vi "Overlay selected point in a miniscan.vi"(8 "error in":errorcluster, 9 "Data reference":refnum<data-value>) -> (0 "error out":errorcluster)   [LabVIEW 2017]
uses:
  xcontrol/Interface VIs/Interface typedefs/Interface-Data array.ctl
  xcontrol/Interface VIs/Interface typedefs/Interface-Data format definition.ctl
  xcontrol/Typedefs/Xctl-XY data type definition.ctl
  xcontrol/Typedefs/Xctrl-ROI type enum.ctl
  Typedefs/Get-Set-Clear Control.ctl
  Global variables/gl_Functional Imaging-Global variables.vi
  xcontrol/XGrapher.xctl
panel:
  in  "Miniscan point overlay colour":u32(colorbox)=16711907
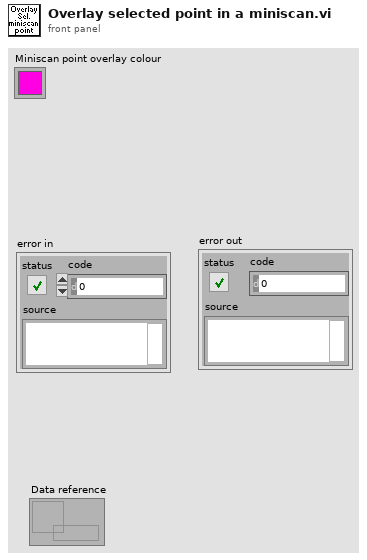
[diagram p1: front panel]
types:
  T1 = typedef "Get-Set-Clear Control.ctl" = enum16{"Get", "Set", "Clear"}
  T2 = typedef "Functional Imging UI Refs.ctl" = cluster{"Menu ref":refnum<k9>, "Image control":refnum<vi>, "VI ref":refnum<vi>, "XGrapher":refnum<vi>, "Smoothing":refnum<vi>, "POI Averaging":refnum<vi>, "Normalize":refnum<vi>, "POI data points in each trial":refnum<vi>, "Channel":refnum<vi>, "Experiment data folder path":refnum<vi>, "[ROI vis]":refnum<vi>, "[Groups] visbl":T3, "Group Name":refnum<vi>, "POI index":refnum<vi>, "Trial No.":refnum<vi>, "Intensity Zoom":refnum<vi>, "Trial Cursor Enabled":refnum<vi>, "Number of Trials (ind 1)":refnum<vi>, "Number of Trials (ind 2)":refnum<vi>, "MiniScans Available":refnum<vi>, "POI Available":refnum<vi>, "Defer graph updates":refnum<vi>, "Waveform selector":refnum<vi>, "#of selected POI":refnum<vi>, "#of selected MiniScans":refnum<vi>, "#of selected groups":refnum<vi>, "Max Z-Projection":refnum<vi>, "Z-Plane Selector":refnum<vi>, "Index of miniscan point to visualise":refnum<vi>, "ROI vis. mode":refnum<vi>, "Total # of points":refnum<vi>, "Index of group clicked on":refnum<vi>, "Pane 1":refnum<vi>, "Pane 2":refnum<vi>, "Pane 3":refnum<vi>, "Pane 4":refnum<vi>, "Pane 5":refnum<vi>, "Pane 6":refnum<vi>, "Deselect all ROI":refnum<vi>, "Deselect all groups":refnum<vi>}
  T3 = typedef "Groups array referecne.ctl" = refnum<vi>
  T4 = typedef "Interface-Data array.ctl" = T5[]
  T5 = typedef "Interface-Data format definition.ctl" = cluster{"Plot.Plot Name":string, "Data":T6, "Timeline data":T6, "Type":T7, "Points per cycle":u16, "ROI number":u16}
  T6 = typedef "XGrapher.xctl/Xctl-XY data type definition.ctl" = cluster{"X-Axis values":sgl[], "Y-Axis values (s)":sgl[]}
  T7 = typedef "Xctrl-ROI type enum.ctl" = enum16{"POI", "Mini-scan", "Group"}
  T8 = typedef "Functional Parameters Cluster.ctl" = cluster{"ROI data":dbl[][], "ROI format version":i32, "Norm ROI data":dbl[][], "Norm. ROI format version":i32, "Z norm":dbl[], "Z norm format version":i32}
  T9 = typedef "ROI parameters data type.ctl" = cluster{"ROI index":dbl, "ROI ID":dbl, "ROI Time (ns)":dbl, "Pixels in ROI":dbl, "X start":dbl, "Y start":dbl, "Z start":dbl, "X stop":dbl, "Y stop":dbl, "Z stop":dbl, "Angle (deg)":dbl, "Composite ID":dbl, "Number of lines":dbl, "Frame Size":dbl, "Zoom":dbl, "Laser Power (%)":dbl, "ROI group ID":dbl}
  T10 = typedef "IMAQ Image.ctl" = refnum<image>
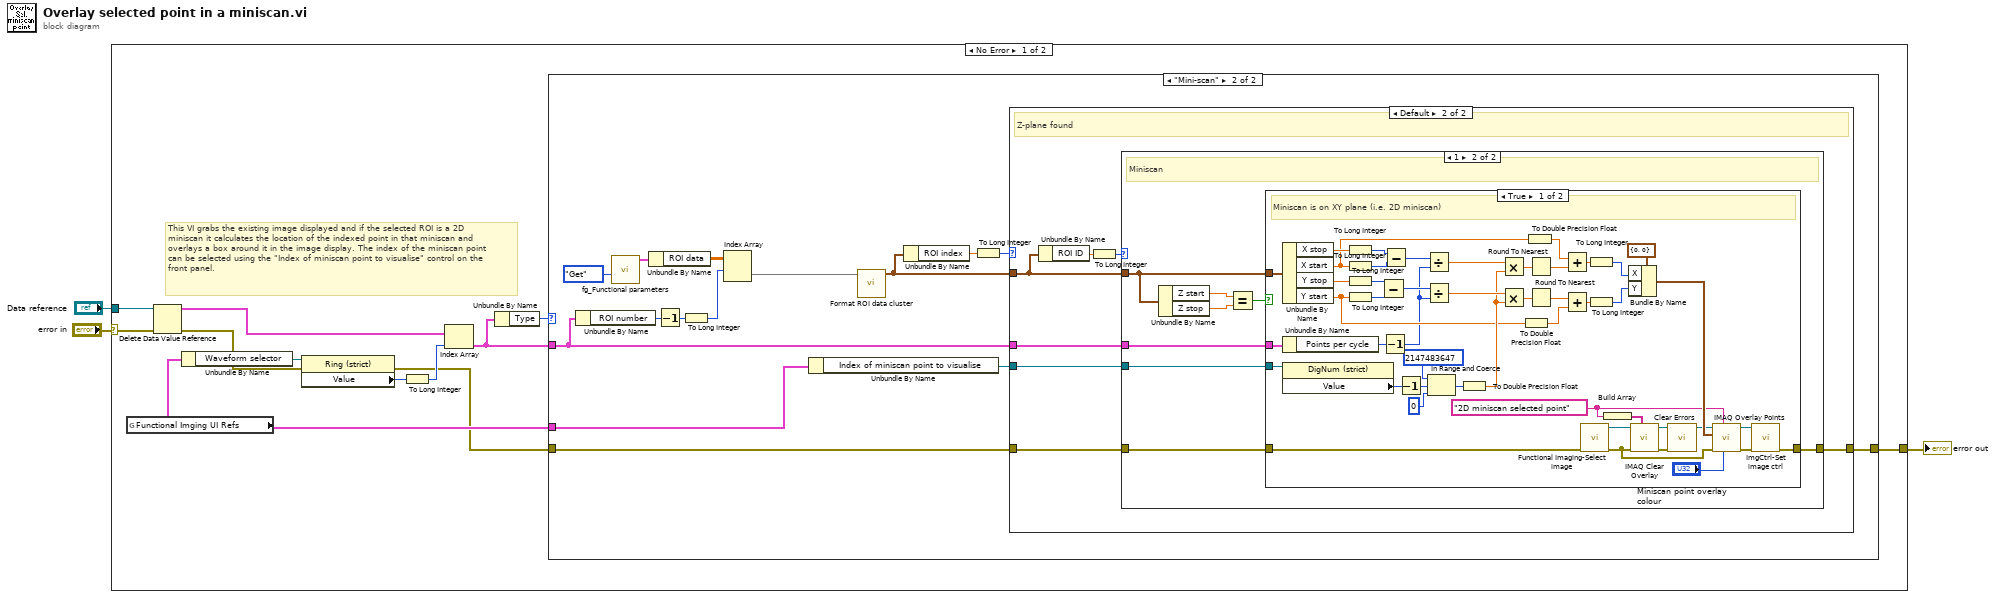
[diagram p0: block diagram]
diagram:
  n1 = case shown="No Error" "error in" {
    selector: "error in" -> [w6 w96]
    tunnel: [w14 w96] -> w3
    tunnel: "Data reference" -> [w8 _]
    frame No Error {
      # "This VI grabs the existing image displayed and if the selected ROI is a 2D miniscan it calculates the location of the indexed point in that miniscan and overlays a box around it in the image display. The index of the miniscan point can be selected using the \"Index of miniscan point to visualise\" control on the front panel."
      n2 = global read "gl_Functional Imaging-Global variables.vi" "Functional Imging UI Refs"() -> (w9:T2)
      n3 = Delete Data Value Reference(data value reference=w8, error in=w6) -> (data value=w7:T4, error out=w5:errorcluster)
      n4 = Unbundle By Name(w9) -> ("Waveform selector"=w11:refnum<vi>)
      n5 = property class="Ring (strict)"(reference=w11, error in=w5) -> (error out=w4:errorcluster, "Value"=w12:u16)  [unwired: 1 out]
      n6 = To Long Integer(number=w12) -> (32bit integer=w13:i32)
      n7 = Index Array(array=w7, index=w13) -> (element=w10:T5)
      n8 = Unbundle By Name(w10) -> ("Type"=w15:T7)
      n9 = case shown="\"Mini-scan\"" w15 {
        tunnel: w9 -> [_ w20]
        tunnel: w10 -> [_ w22]
        tunnel: [w16 w21] -> w14
        tunnel: w4 -> [w16 w17]
        frame Default {
        }
        frame "Mini-scan" {
          n10 = Unbundle By Name(w22) -> ("ROI number"=w23:u16)
          n11 = call "fg_Functional parameters.vi"("Function"=Get-Set-Clear_Control."Get") -> ("Functional Parameters"=w31:T8)  [unwired: 7 in, 3 out]
          n12 = Unbundle By Name(w31) -> ("ROI data"=w29:dbl[][])
          n13 = Decrement(x=w23) -> (x-1=w28:u16)
          n14 = To Long Integer(number=w28) -> (32bit integer=w26:i32)
          n15 = Index Array(array=w29, index (row)=w26) -> (element=w27:dbl[])  [unwired: 1 in]
          n16 = Unbundle By Name(w20) -> ("Index of miniscan point to visualise"=w19:refnum<vi>)
          n17 = call "Format ROI data cluster.vi"("Single ROI info"=w27) -> ("X-Y-Z coordinates"=w24:T9)  [unwired: 10 in]
          n18 = Unbundle By Name(w24) -> ("ROI index"=w25:dbl)
          n19 = To Long Integer(number=w25) -> (32bit integer=w18:i32)
          n20 = case shown="Default" w18 {
            tunnel: w24 -> [_ w38]
            tunnel: w22 -> [_ w37]
            tunnel: [w32 w36] -> w21
            tunnel: w19 -> [_ w35]
            tunnel: w17 -> [w32 w33]
            frame -1 {
              # "Z-plane not found"
            }
            frame Default {
              # "Z-plane found"
              n21 = Unbundle By Name(w38) -> ("ROI ID"=w39:dbl)
              n22 = To Long Integer(number=w39) -> (32bit integer=w34:i32)
              n23 = case shown="1" w34 {
                tunnel: w38 -> [_ w45]
                tunnel: w37 -> [_ w44]
                tunnel: [w40 w43] -> w36
                tunnel: w35 -> [_ w42]
                tunnel: w33 -> [w40 w41]
                frame Default {
                  # "Unsupported ROI type"
                }
                frame 1 {
                  # "Miniscan"
                  n24 = Unbundle By Name(w45) -> ("Z start"=w48:dbl, "Z stop"=w47:dbl)
                  n25 = Equal?(x=w48, y=w47) -> (x = y?=w46:bool)
                  n26 = case shown="True" w46 {
                    tunnel: w45 -> [w91 _]
                    tunnel: w44 -> [w89 _]
                    tunnel: [w50 w95] -> w43
                    tunnel: w42 -> [w71 _]
                    tunnel: w41 -> [w49 w95]
                    frame True {
                      w56 = "2D miniscan selected point" ("Group")
                      # "Miniscan is on XY plane (i.e. 2D miniscan)"
                      n27 = Unbundle By Name(w91) -> ("X stop"=w92:dbl, "X start"=w66:dbl, "Y stop"=w93:dbl, "Y start"=w65:dbl)
                      n28 = Unbundle By Name(w89) -> ("Points per cycle"=w82:u16)
                      n29 = property on="Property Node" class="DigNum (strict)"(reference=w71) -> ("Value"=w79:i32)  [unwired: 1 in, 2 out]
                      n30 = To Long Integer(number=w92) -> (32bit integer=w87:i32)
                      n31 = To Long Integer(number=w66) -> (32bit integer=w69:i32)
                      n32 = To Long Integer(number=w93) -> (32bit integer=w86:i32)
                      n33 = To Long Integer(number=w65) -> (32bit integer=w85:i32)
                      n34 = Subtract(x=w86, y=w85) -> (x-y=w83:i32)
                      n35 = Decrement(x=w82) -> (x-1=w57:u16)
                      n36 = Subtract(x=w87, y=w69) -> (x-y=w84:i32)
                      n37 = Decrement(x=w79) -> (x-1=w78:i32)
                      n38 = Divide(x=w84, y=w57) -> (x/y=w81:dbl)
                      n39 = Divide(x=w83, y=w57) -> (x/y=w80:dbl)
                      n40 = In Range and Coerce(upper limit=2147483647, x=w78, lower limit=0) -> (coerced(x)=w77:i32)  [unwired: 1 out]
                      n41 = To Double Precision Float(number=w77) -> (double precision float=w72:dbl)
                      n42 = Multiply(x=w81, y=w72) -> (x*y=w74:dbl)
                      n43 = Multiply(x=w80, y=w72) -> (x*y=w73:dbl)
                      n44 = To Double Precision Float(number=w65) -> (double precision float=w64:dbl)
                      n45 = To Double Precision Float(number=w66) -> (double precision float=w67:dbl)
                      n46 = Round To Nearest(number=w74) -> (nearest integer value=w70:dbl)
                      n47 = Round To Nearest(number=w73) -> (nearest integer value=w63:dbl)
                      n48 = Add(x=w67, y=w70) -> (x+y=w68:dbl)
                      n49 = Add(x=w63, y=w64) -> (x+y=w62:dbl)
                      n50 = call "Functional Imaging-Select image.vi"("error in (no error)"=w49) -> ("error out"=w59:errorcluster, "SelectedPOIMax"=w53:T10)  [unwired: 9 in]
                      n51 = To Long Integer(number=w68) -> (32bit integer=w55:i32)
                      n52 = To Long Integer(number=w62) -> (32bit integer=w54:i32)
                      n53 = Build Array(w56) -> (w60:string[])
                      n54 = Bundle By Name(cluster=cluster{"X":i32, "Y":i32} {"X"=0, "Y"=0} ("Point"), "X"=w55, "Y"=w54) -> (w88:cluster{"X":i32, "Y":i32})
                      n55 = call "IMAQ Clear Overlay"("Groups"=w60, "error in (no error)"=w59, "Image"=w53) -> ("error out"=w58:errorcluster, "Image Out"=w61:T10)  [unwired: 7 in]
                      n56 = call <vilib>:"Clear Errors.vi"("error in (no error)"=w58) -> ()  [unwired: 5 in, 2 out]
                      n57 = call "IMAQ Overlay Points"("Color"="Miniscan point overlay colour", "Group"=w56, "error in (no error)"=w59, "Point"=w88, "Image"=w61) -> ("error out"=w51:errorcluster, "Image Out"=w52:T10)  [unwired: 5 in]
                      n58 = call "ImgCtrl-Set image ctrl.vi"("error in"=w51, "Image"=w52) -> ("error out"=w50:errorcluster)  [unwired: 9 in]
                    }
                    frame False {
                      # "I don't believe this functionality could be applied to 3D miniscans"
                      # "3D miniscan"
                    }
                  }
                }
              }
            }
          }
        }
      }
    }
    frame Error {
    }
  }
  "error out" <- w3
